vi "After Each.vi"(8 "Error In":errorcluster, 11 "Writer In":refnum<class "Writer.lvclass">) -> (0 "Error Out":errorcluster, 3 "Data":string)   [LabVIEW 2017, in "Tests.lvlib" / "Writer.lvlib"]
uses:
  Writer.lvlib
  src/LabPack/Public/Writer/Writer.lvclass
  src/LabPack/Public/Writer/Private/End by Value.vi
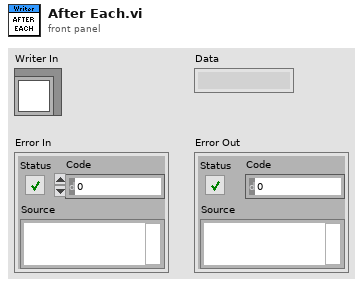
[diagram p1: front panel]
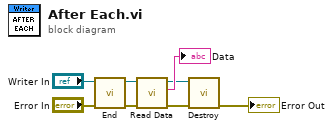
[diagram p0: block diagram]
diagram:
  n1 = call-poly "End.vi"("Error In"="Error In", "Writer In"="Writer In") -> ("Error Out"=w5:errorcluster, "Writer Out"=w4:refnum<class "Writer.lvclass">)  [unwired: 8 in]
  n2 = call "Read Data.vi"("Error In"=w5, "Writer In"=w4) -> ("Error Out"=w6:errorcluster, "Data"=→"Data":string, "Writer Out"=w7:refnum<class "Writer.lvclass">)  [unwired: 7 in]
  n3 = call "Destroy.vi"("Error In"=w6, "Writer"=w7) -> ("Error Out"=→"Error Out":errorcluster)  [unwired: 9 in]
